vi "Assert Array Empty.vi"(4 "Execution time (s)":dbl=-1.0, 5 "Assert Only? (F)":bool, 6 "error code (1)":i32=1, 7 "Label (\"\")":string, 8 "error in (no error)":errorcluster, 9 "Register with caller test (F)":bool, 11 "Array":variant) -> (0 "error out":errorcluster, 2 "Properties.Assert":refnum<class "Properties.Assert.lvclass">)   [LabVIEW 2013, in "Caraya.lvlib" / "Assert.lvclass"]
doc: "Asserts that an array is empty."
uses:
  Assert.lvclass
  Properties.Assert/Properties.Assert.lvclass
  Properties/Properties.lvclass
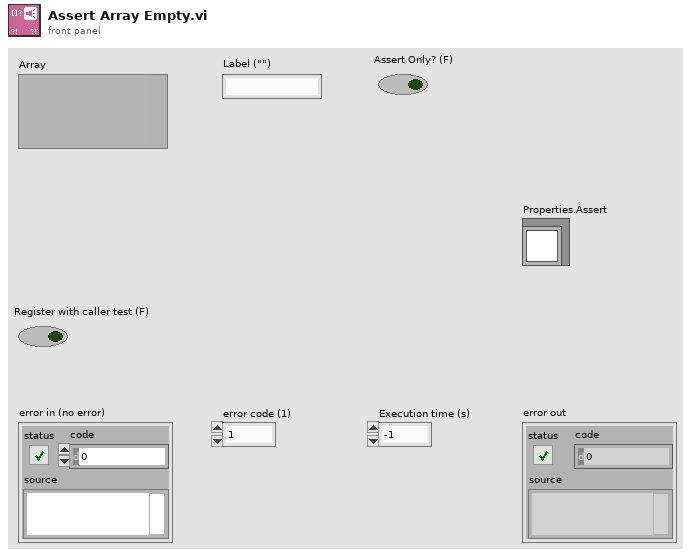
[diagram p1: front panel]
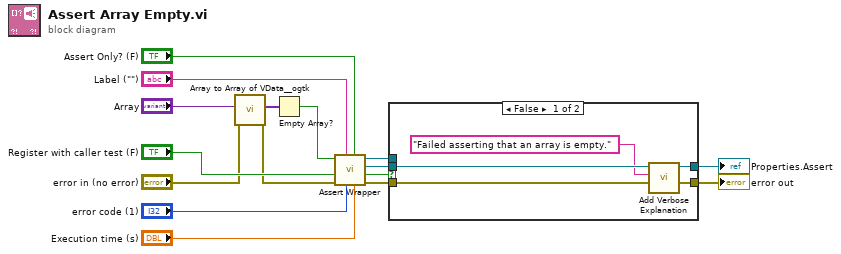
[diagram p0: block diagram]
diagram:
  n1 = call <userlib>:"Array to Array of VData__ogtk.vi"("error in (no error)"="error in (no error)", "MultiD Array"="Array") -> ("error out"=w3:errorcluster, "1D Array of Variants"=w2:variant[])  [unwired: 8 in]
  n2 = Empty Array?(array=w2) -> (empty?=w1:bool)
  n3 = call "Assert Wrapper.vi"("Execution time (s)"="Execution time (s)", "Assert Only? (F)"="Assert Only? (F)", "error code (1)"="error code (1)", "Label"="Label (\"\")", "error in (no error)"=w3, "Register with caller test (F)"="Register with caller test (F)", "Assert?"=w1) -> ("error out"=w7:errorcluster, "Verbose"=w11:bool, "Properties.Assert"=w9:refnum<class "Properties.Assert.lvclass">, "Assert out"=w10:refnum<class "Assert.lvclass">)  [unwired: 1 in]
  n4 = case shown="False" w11 {
    tunnel: w10 -> [_ _]
    tunnel: w9 -> [w19 w23]
    tunnel: [w20 w22] -> w8
    tunnel: w7 -> [w21 w22]
    tunnel: [w18 w23] -> w6
    frame False {
      n5 = call "Add Verbose Explanation.vi"("error in (no error)"=w21, "Verbose Explanation"="Failed asserting that an array is empty.", "Properties"=w19) -> ("error out"=w20:errorcluster, "Properties"=w18:refnum<class "Properties.Assert.lvclass">)  [unwired: 7 in]
    }
    frame True {
    }
  }
  "error out" <- w8
  "Properties.Assert" <- w6
